vi "时间-温度曲线(子VI).vi"   [LabVIEW 2016, in "斯坦道CODMn新电路板.lvlib"]
uses:
  <vilib>/ptbypt/NI_PtbyPt.lvlib
types:
  T1 = enum16{"空闲", "水样测试", "标样核查", "零点核查", "跨度核查", "空白测试", "平行样测试", "加标回收", "空白校准", "标样校准", "初始化（清洗）"}
  T2 = cluster{"系统时间":timestamp, "工作状态":u16, "测量模式":enum16{"待机", "连续模式", "周期模式", "定点模式", "受控模式", "手动模式"}, "告警代码":u16, "故障代码":u16, "日志代码":u16, "软件版本":u16, "A":sgl, "B":sgl, "K":sgl, "当前滴定数":sgl, "T":sgl, "H":sgl, "id":u16, "flowid":u16, "量程":u16, "加热实时温度":sgl, "当前ORP值":sgl, "运行时间":sgl, "当前步骤剩余时间":sgl, "结束滴定数":sgl, "注射泵保温温度":sgl, "匹配滴定数X0":u16, "X^2":sgl, "X":sgl, "B 2":sgl, "光值1":sgl, "光值2":sgl, "光值3":sgl, "光值4":sgl, "光值5":sgl, "光值6":sgl, "光值7":sgl, "光值8":sgl}
  T3 = typedef "工况数据.ctl" = cluster{"time":string, "data":cluster{"ups":cluster{"ups":cluster{"input_voltage":ext, "input_frequency":ext, "output_voltage":ext, "output_current":ext, "output_frequency":ext, "output_active_power":ext, "output_apparent_power":ext, "load_rate":ext, "cabinet_temperature":ext, "battery_voltage":ext, "remaining_battery_capacity":ext, "power_on_status":string, "power_supply_mode":string, "fault":bool, "battery_low_voltage":bool, "mains_supply_abnormality":bool}, "启用":bool}, "air_conditioner":cluster{"air_conditioner":cluster{"cabinet_temperature":ext, "air_supply_temperature":ext, "voltage":ext, "current":ext, "compressor_status":string, "Internal_fan_status":string, "external_fan_status":string, "heating_state":string, "refrigeration_state":bool, "high_temperature_alarm":bool, "low_temperature_alarm":bool, "heater_fault":bool, "temperature_sensor_fault":bool, "high_voltage_alarm":bool, "low_voltage_alarm":bool, "refrigeration_start_point":ext, "refrigeration_sensitive_point":ext, "heating_start_point":ext, "heating_sensitive_point":ext, "high_temperature_alarm_point":ext, "low_temperature_alarm_point":ext}, "启用":bool}, "smoke_sensor":cluster{"smoke_sensor":cluster{"trigger_alarm":bool}, "启用":bool}, "water_immersion_sensor":cluster{"water_immersion_sensor":cluster{"trigger_alarm":bool}, "启用":bool}, "temperature_and_humidity_sensor":cluster{"temperature_and_humidity_sensor":cluster{"current_temperature":ext, "current_humidity":ext, "room_temperature_alarm":bool, "humidity_alarm":bool}, "启用":bool}, "gps":cluster{"gps":cluster{"current_longitude":ext, "current_latitude":ext, "launch_longitude":ext, "launch_latitude":ext, "shift_alarm":bool}, "启用":bool}, "solar_controller":cluster{"solar_controller":cluster{"array_voltage":ext, "array_current":ext, "generating_power":ext, "battery_voltage":dbl, "battery_current":ext, "ceiling_voltage":ext, "minimum_voltage":ext, "battery_temperature":ext, "remaining_battery_capacity":ext, "load_voltage":ext, "load_current":ext, "load_power":ext, "equipment_temperature":ext, "accumulated_electricity_consumption_of_the_day":ext, "accumulated_electricity_consumption_of_the_current_month":ext, "accumulated_electricity_consumption_in_the_current_year":ext, "total_accumulated_power_consumption":ext, "accumulated_charging_capacity_of_the_day":ext, "accumulated_charging_amount_of_the_current_month":ext, "accumulated_charging_capacity_of_the_current_year":ext, "total_cumulative_charge":ext}, "启用":bool}, "solar_controller_2":cluster{"solar_controller_2":cluster{"array_voltage":ext, "array_current":ext, "generating_power":ext, "battery_voltage":dbl, "battery_current":ext, "ceiling_voltage":ext, "minimum_voltage":ext, "battery_temperature":ext, "remaining_battery_capacity":ext, "load_voltage":ext, "load_current":ext, "load_power":ext, "equipment_temperature":ext, "accumulated_electricity_consumption_of_the_day":ext, "accumulated_electricity_consumption_of_the_current_month":ext, "accumulated_electricity_consumption_in_the_current_year":ext, "total_accumulated_power_consumption":ext, "accumulated_charging_capacity_of_the_day":ext, "accumulated_charging_amount_of_the_current_month":ext, "accumulated_charging_capacity_of_the_current_year":ext, "total_cumulative_charge":ext}, "启用":bool}, "NH3":cluster{"NH3":cluster{"F0":ext, "F1":ext, "syringe_temperature":ext, "alarm_step":dbl, "X0":ext}, "启用":bool}, "TP":cluster{"TP":cluster{"F0":ext, "F1":ext, "F2":ext, "F3":ext, "digestion_temperature":ext, "constant_temperature":ext, "syringe_temperature":ext, "alarm_step":dbl, "X0":ext}, "启用":bool}, "TN":cluster{"TN":cluster{"F0":ext, "F1":ext, "F2":ext, "F3":ext, "F4":ext, "F5":ext, "F6":ext, "F7":ext, "digestion_temperature":ext, "constant_temperature":ext, "syringe_temperature":ext, "alarm_step":dbl, "X0":ext}, "启用":bool}, "CODMn":cluster{"CODMn":cluster{"temperature_curve":ext[], "titration_curve":ext[], "F0":ext, "F1":ext, "F2":ext, "F3":ext, "F4":ext, "F5":ext, "A":ext, "B":ext, "K":ext}, "启用":bool}, "CODCr":cluster{"CODCr":cluster{"temperature_curve":ext[], "F0":ext, "F1":ext, "reagent_sensor":ext}, "启用":bool}}}
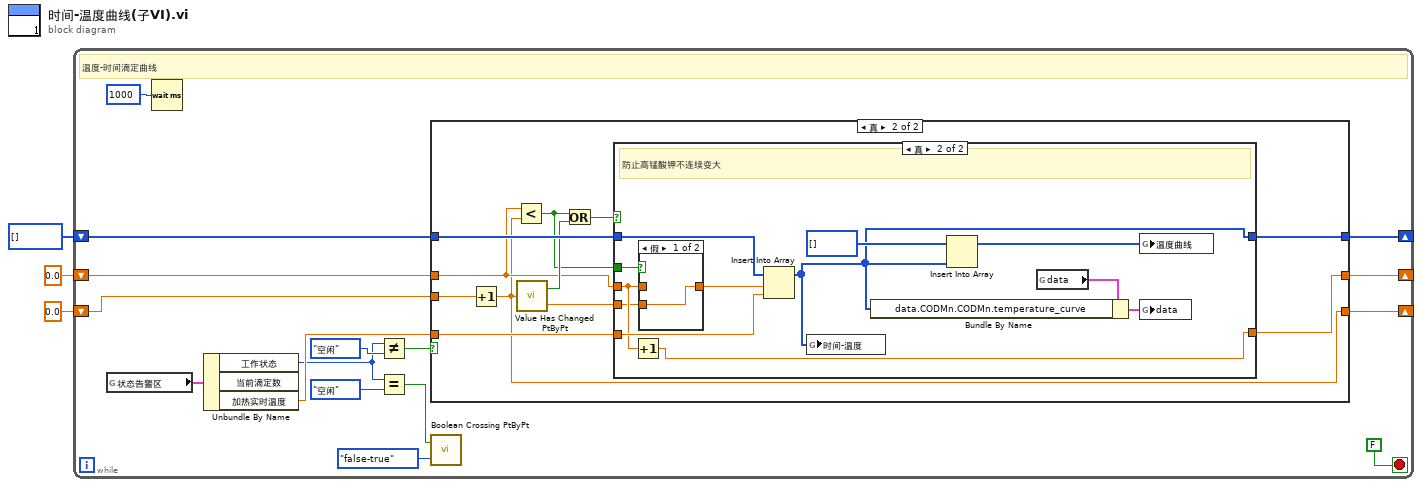
[diagram p0: block diagram]
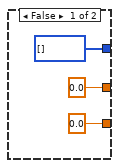
[diagram p2: hidden frame]
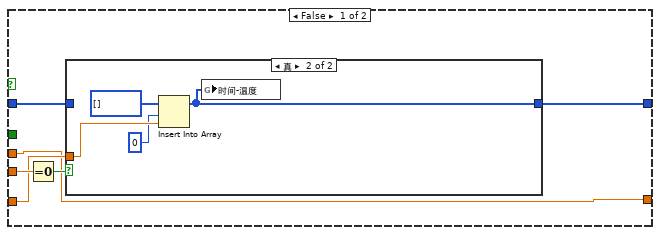
[diagram p3: hidden frame]
diagram:
  n1 = while {
    shift-right: [w16] -> _
    shift-left: u16[] [] ("ORP滴定曲线") -> [w17]
    shift-right: [w14] -> _
    shift-left: 0.0 -> [w15]
    shift-right: [w4] -> _
    shift-left: 0.0 -> [w5]
    stop <- FALSE stop-if-true
    # "温度-时间滴定曲线"
    n2 = global read "VARCODMn全局变量.vi" "状态告警区"() -> (w13:T2)
    n3 = Wait (ms)(milliseconds to wait=u32 1000 ("等待时间（毫秒）")) -> ()  [unwired: 1 out]
    n4 = Unbundle By Name(w13) -> ("工作状态"=w6:u16, "加热实时温度"=w10:sgl)  [unwired: 1 out]
    n5 = Not Equal?(x=w6, y=T1."空闲" ("工作状态")) -> (x != y?=w11:bool)
    n6 = Equal?(x=w6, y=T1."空闲" ("工作状态")) -> (x = y?=w8:bool)
    n7 = case shown="真" w11 {
      tunnel: w17 -> [_ w33]
      tunnel: [u16[] [] ("ORP滴定曲线") w32] -> w16
      tunnel: w15 -> [_ w28]
      tunnel: [0.0 w27] -> w14
      tunnel: w10 -> [_ w25]
      tunnel: w5 -> [_ w24]
      tunnel: [0.0 w23] -> w4
      frame False {
      }
      frame True {
        n8 = Increment(x=w24) -> (x+1=w23:dbl)
        n9 = Less?(x=w28, y=w23) -> (x < y?=w26:bool)
        n10 = call <vilib>:"Value Has Changed PtByPt.vi"("input data point"=w23) -> ("has changed"=w31:bool, "output data point"=w30:dbl)  [unwired: 1 in]
        n11 = Or(x=w26, y=w31) -> (x .or. y?=w29:bool)
        n12 = case shown="真" w29 {
          tunnel: w33 -> [w38 w55]
          tunnel: [w37 w45] -> w32
          tunnel: w30 -> [w39 w49]
          tunnel: w25 -> [w35 w54]
          tunnel: w28 -> [w34 w51]
          tunnel: [w34 w53] -> w27
          tunnel: w26 -> [_ w52]
          frame False {
            n13 = Equal To 0?(x=w39) -> (x = 0?=w36:bool)
            n14 = case shown="真" w36 {
              tunnel: [w40 w41] -> w37
              tunnel: w38 -> [w40 _]
              tunnel: w35 -> [_ w43]
              frame False {
              }
              frame True {
                n15 = Insert Into Array(array=u16[] [] ("ORP滴定曲线"), index=0 ("索引"), new element=w43) -> (w41:u16[])
                n16 = global write "VARCODMn全局变量.vi" "时间-温度"(w41) -> ()
              }
            }
          }
          frame True {
            # "防止高锰酸钾不连续变大"
            n17 = Increment(x=w51) -> (x+1=w53:dbl)
            n18 = case shown="假" w52 {
              tunnel: w51 -> [_ w58]
              tunnel: [w57 w58] -> w50
              tunnel: w49 -> [w57 _]
              frame False {
              }
              frame True {
              }
            }
            n19 = Insert Into Array(array=w55, index=w50, new element=w54) -> (w45:u16[])
            n20 = global write "VARCODMn全局变量.vi" "时间-温度"(w45) -> ()
            n21 = Insert Into Array(array=u16[] [] ("ORP滴定曲线"), new element=w45) -> (w48:u16[])  [unwired: 1 in]
            n22 = global read "工况数据接口全局.vi" "data"() -> (w46:T3)
            n23 = Bundle By Name(cluster=w46, "data.CODMn.CODMn.temperature_curve"=w45) -> (w47:T3)
            n24 = global write "VARCODMn全局变量.vi" "温度曲线"(w48) -> ()
            n25 = global write "工况数据接口全局.vi" "data"(w47) -> ()
          }
        }
      }
    }
    n26 = call <vilib>:"Boolean Crossing PtByPt.vi"("direction"=enum16{"either", "false-true", "true-false"}."false-true", "input"=w8) -> ()  [unwired: 1 in, 1 out]
  }
